vi "TDMS Initial.vi"(8 "error in":errorcluster, 11 "AOL_Globals":T1={"Imaging Protocol"=enum."AOL Z-Stack", "Number of POI"=0, "Number of Miniscans"=0, "Number of Trials"=0, "Number of Cycles "=0, "# Averaged Frames"=0, "Laser power (%)"=0, "Pockels"=0.0, "Acquisition Length (sec)"=0.0, "Fill time (us)"=0.0, "POI Dwell time (us)"=0.0, "Miniscan Dwell time per pixel (us)"=0.0, "PMT 1"=0.0, "PMT 2"=0.0, "Back Apperture"=0.0, "Frame Size"=0, "Center Frequency"=0.0, "Field of View"=0.0, "DwellTime (us)"=0.0, "Wavelength (nm)"=0.0, "Zoom"=0.0, "AOL Z"=0.0, "AOL Mode"=enum."Raster", "GridXY"=0.0, "GridZ"=0.0, "TriggerPeriod (sec)"=0.0, "Number of Pixels in Miniscan"=0, "Experiment folder path"=path "", "X centre"=0.0, "Y centre"=0.0, "Angle (degrees)"=0.0, "Plane Mode"=0, "Threshold"=[], "Regenerate Chirps"=FALSE, "Rectangle ROI length (pixels)"=0, "Rectangle ROI height (pixels)"=0, "AOD fill"=0, "Samples Wait after Trigger"=0, "StartUp Delay"=0, "Slip Cycle"=163840, "Add Cycle"=FALSE} {"Plane Mode" items=["XY Plane"]; "Frame Size" items=["100X100"=100, "128X128"=128, "200X200"=200, "256X256"=256, "512X512"=512, "1024x1024"=1024, "2048x2048"=2048]; "Back Apperture" format="%#.6g"; "Pockels" format="%#.6g"; "PMT 2" format="%#.6g"; "PMT 1" format="%#.6g"; "Angle (degrees)" format="%#.6g"; "POI Dwell time (us)" format="%#.6g"}) -> (0 "error IO":errorcluster, 2 "TDMS file paths OR experiment folder path":path[](array[path]), 3 "Functional imaging TDMS file references":refnum<k34>[](array[refnum]))   [LabVIEW 2013]
uses:
  Typedefs/Controls/AOL_Globals.ctl
  Typedefs/Imaging Protocols enum.ctl
  Typedefs/Frame Size.ctl
  Typedefs/AOL modes.ctl
  Typedefs/Plane Mode.ctl
  Global Variables/General Globals.vi
panel:
  in  "disable buffering (T)":bool
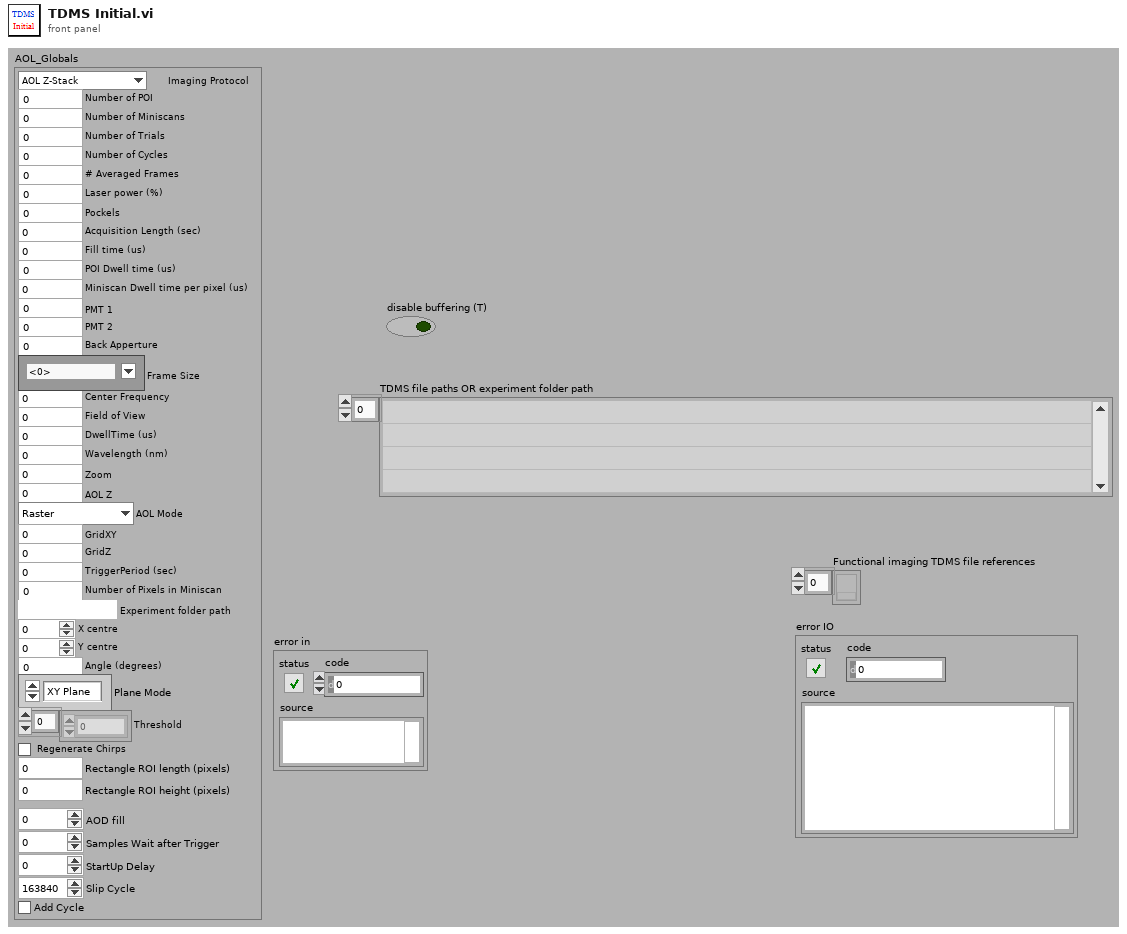
[diagram p1: front panel]
types:
  T1 = typedef "AOL_Globals.ctl" = cluster{"Imaging Protocol":T2, "Number of POI":u16, "Number of Miniscans":u16, "Number of Trials":u16, "Number of Cycles ":u64, "# Averaged Frames":u16, "Laser power (%)":u8, "Pockels":dbl, "Acquisition Length (sec)":dbl, "Fill time (us)":dbl, "POI Dwell time (us)":dbl, "Miniscan Dwell time per pixel (us)":dbl, "PMT 1":dbl, "PMT 2":dbl, "Back Apperture":dbl, "Frame Size":T3, "Center Frequency":dbl, "Field of View":dbl, "DwellTime (us)":dbl, "Wavelength (nm)":dbl, "Zoom":dbl, "AOL Z":dbl, "AOL Mode":T4, "GridXY":dbl, "GridZ":dbl, "TriggerPeriod (sec)":dbl, "Number of Pixels in Miniscan":u16, "Experiment folder path":path, "X centre":dbl, "Y centre":dbl, "Angle (degrees)":dbl, "Plane Mode":T5, "Threshold":u16[], "Regenerate Chirps":bool, "Rectangle ROI length (pixels)":u16, "Rectangle ROI height (pixels)":u16, "AOD fill":u16, "Samples Wait after Trigger":u16, "StartUp Delay":i32, "Slip Cycle":u32, "Add Cycle":bool}
  T2 = typedef "Imaging Protocols enum.ctl" = enum16{"AOL Z-Stack", "Motor Z Stack", "Functional Acquisition", "Single Plane Acquisition", "Volume Acquisition", "Live Imaging", "Live Plane Imaging", "Live Volume Imaging"}
  T3 = typedef "Frame Size.ctl" = u16
  T4 = typedef "AOL modes.ctl" = enum16{"Raster", "Structural", "Pointing", "Mini Scan", "Alignment"}
  T5 = typedef "Plane Mode.ctl" = u16
  T6 = enum16{"open", "open or create", "create or replace", "create", "open (read-only)"}
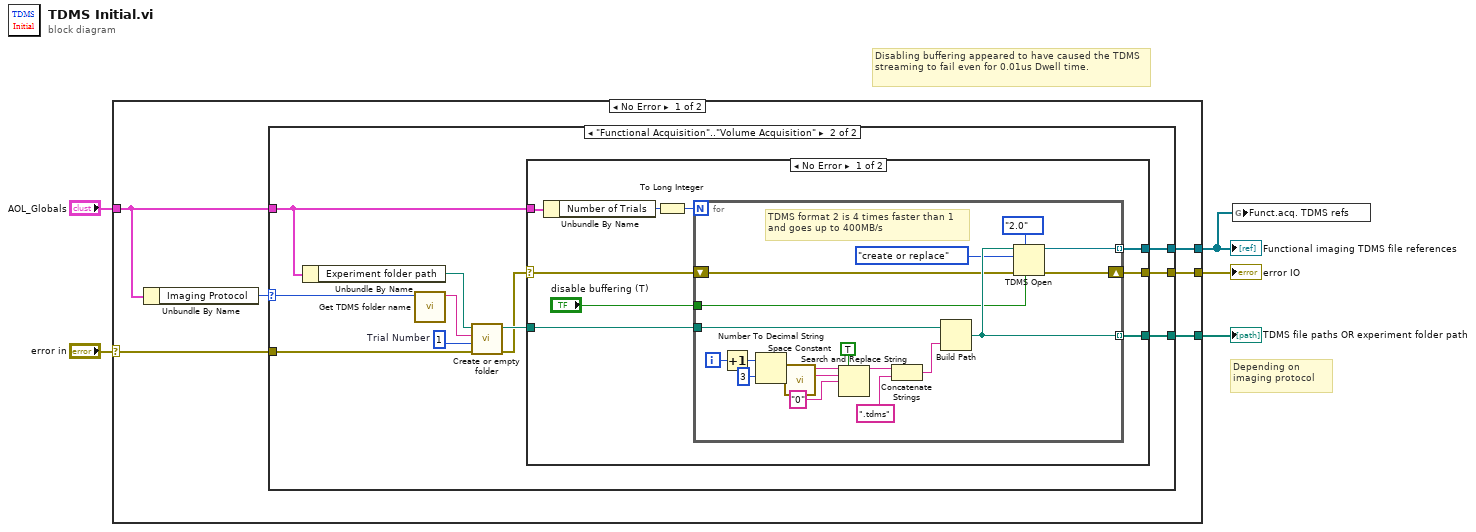
[diagram p0: block diagram]
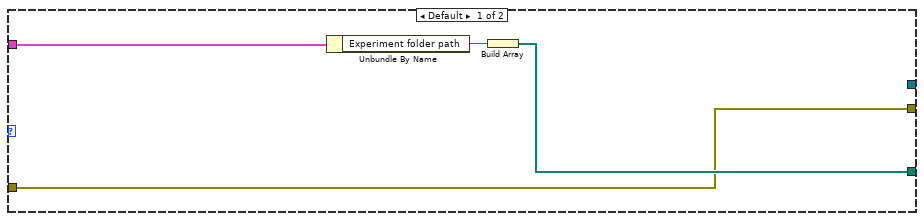
[diagram p2: hidden frame]
diagram:
  # "Disabling buffering appeared to have caused the TDMS streaming to fail even for 0.01us Dwell time."
  # "Depending on imaging protocol"
  n1 = case shown="No Error" "error in" {
    selector: "error in" -> [w6 w55]
    tunnel: [w11 _] -> w1
    tunnel: [w10 _] -> w5
    tunnel: [w9 w55] -> w4
    tunnel: "AOL_Globals" -> [w7 _]
    frame No Error {
      n2 = Unbundle By Name(w7) -> ("Imaging Protocol"=w8:T2)
      n3 = case shown="\"Functional Acquisition\"..\"Volume Acquisition\"" w8 {
        selector: w8 -> [_ w16]
        tunnel: [_ w26] -> w11
        tunnel: w7 -> [w13 w18]
        tunnel: [w15 w25] -> w10
        tunnel: [w14 w23] -> w9
        tunnel: w6 -> [w14 w21]
        frame Default {
          n4 = Unbundle By Name(w13) -> ("Experiment folder path"=w12:path)
          n5 = Build Array(w12) -> (w15:path[])
        }
        frame "Functional Acquisition".."Volume Acquisition" {
          w22 = 1  # Trial Number
          n6 = Unbundle By Name(w18) -> ("Experiment folder path"=w19:path)
          n7 = call "Get TDMS folder name.vi"("Imaging Protocol"=w16) -> ("TDMS files folder name"=w17:string)  [unwired: 10 in]
          n8 = call "Create or empty folder.vi"("error in (no error)"=w21, "Trial Number"=w22, "name of folder to create or empty"=w17, "Experiment folder path"=w19) -> ("error out"=w20:errorcluster, "appended path"=w24:path)  [unwired: 6 in]
          n9 = case shown="No Error" w20 {
            selector: w20 -> [w32 w54]
            tunnel: [w35 _] -> w26
            tunnel: w18 -> [w28 _]
            tunnel: [w34 _] -> w25
            tunnel: w24 -> [w33 _]
            tunnel: [w31 w54] -> w23
            frame No Error {
              n10 = Unbundle By Name(w28) -> ("Number of Trials"=w30:u16)
              n11 = To Long Integer(number=w30) -> (32bit integer=w29:i32)
              n12 = for {
                N: w29 -> [_]
                tunnel: [w51] -> w35 mode=indexing
                tunnel: [w49] -> w34 mode=indexing
                tunnel: w33 -> [w40]
                shift-right: [w39] -> w31
                shift-left: w32 -> [w38]
                tunnel: "disable buffering (T)" -> [w37]
                i -> [w50]
                # "TDMS format 2 is 4 times faster than 1\nand goes up to 400MB/s"
                n13 = Increment(x=w50) -> (x+1=w44:i32)
                n14 = Number To Decimal String(number=w44, width (-)=i16 3) -> (decimal integer string=w47:string)
                n15 = call <vilib>:"Space Constant.vi"() -> ("String"=w43:string)
                n16 = Search and Replace String(replace all?=TRUE ("replace all? (F)"), input string=w47, search string=w43, replace string="0" ("replace string (\"\")")) -> (result string=w46:string)  [unwired: 4 in, 3 out]
                n17 = Concatenate Strings(w46, ".tdms" ("string")) -> (w48:string)
                n18 = Build Path(base path=w40, name or relative path=w48) -> (appended path=w49:path)
                n19 = TDMS Open(6:w37, 7:enum16{"1.0", "2.0"}."2.0" ("file format version (2.0)"), 8:w38, 10:T6."create or replace" ("operation (0:open)"), 11:w49) -> (0:w39:errorcluster, 3:w51:refnum<k34>)  [unwired: 2 in]
              }
            }
            frame Error {
            }
          }
        }
      }
    }
    frame Error {
    }
  }
  "Functional imaging TDMS file references" <- w1
  "TDMS file paths OR experiment folder path" <- w5
  "error IO" <- w4
  n20 = global write "General Globals.vi" "Funct.acq. TDMS refs"(w1) -> ()
